vi "Gen - Computer ID.vi"(8 "Error In":errorcluster, 11 "Path":string="C:\\Program Files (x86)\\National Instruments\\Shared\\License Manager\\bin\\generateComputerId.exe") -> (0 "Error Out":errorcluster, 3 "COMPUTER ID":string)   [LabVIEW 2020]
doc: "This VI use to run generateComputerId.exe and generate computer ID.\nPath: path of generateComputerId.exe"
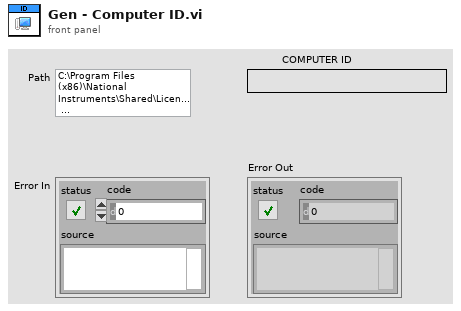
[diagram p1: front panel]
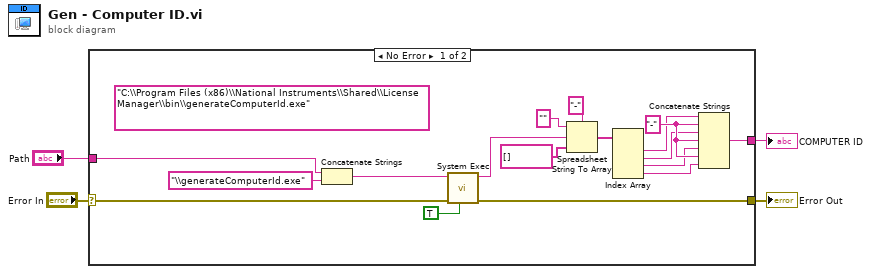
[diagram p0: block diagram]
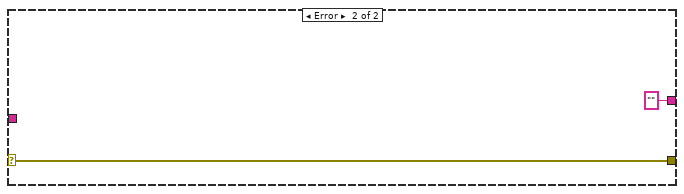
[diagram p2: hidden frame]
diagram:
  n1 = case shown="No Error" "Error In" {
    selector: "Error In" -> [w21 w23]
    tunnel: [w20 w23] -> w3
    tunnel: "Path" -> [w19 _]
    tunnel: [w7 ""] -> w1
    frame No Error {
      (unwired) "C:\\Program Files (x86)\\National Instruments\\Shared\\License Manager\\bin\\generateComputerId.exe" ("command line")
      w14 = "-" ("delimiter (Tab)")
      n2 = Concatenate Strings(w19, "\\generateComputerId.exe" ("string")) -> (w6:string)
      n3 = call <vilib>:"System Exec.vi"("run minimized? (F)"=TRUE, "error in (no error)"=w21, "command line"=w6) -> ("error out"=w20:errorcluster, "standard output"=w17:string)  [unwired: 5 in, 2 out]
      n4 = Spreadsheet String To Array(delimiter (Tab)="-", format string="" ("string"), spreadsheet string=w17, array type (2D Dbl)=string[] []) -> (array=w9:string[])
      n5 = Index Array(array=w9) -> (element #1=w13:string, element #2=w12:string, element #3=w11:string, element #4=w10:string)  [unwired: 4 in]
      n6 = Concatenate Strings(w13, w14, w12, w14, w11, w14, w10) -> (w7:string)
    }
    frame Error {
    }
  }
  "COMPUTER ID" <- w1
  "Error Out" <- w3
